vi "FTW-Connector-SendPoisonPill.vi"(0 "FTW Actor Connector":refnum<class "FTW-ActorConnector.lvclass">, 5 "Timeout":i32=100 format="%dmsec", 11 "error in":errorcluster) -> (4 "FTW Actor Connector out":refnum<class "FTW-ActorConnector.lvclass">, 6 "Response Header":string, 8 "Response Body":string, 10 "Timed out?":bool, 15 "error out":errorcluster)   [LabVIEW 2013, in "FTW-Actor.lvlib" / "FTW-ActorConnector.lvclass"]
uses:
  FTW-ActorConnector.lvclass
panel:
  # "Inputs"
  # "Outputs"
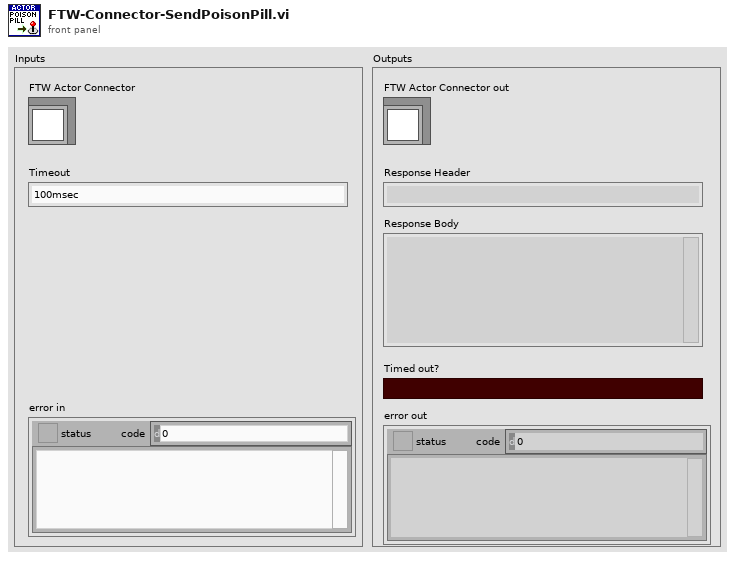
[diagram p1: front panel]
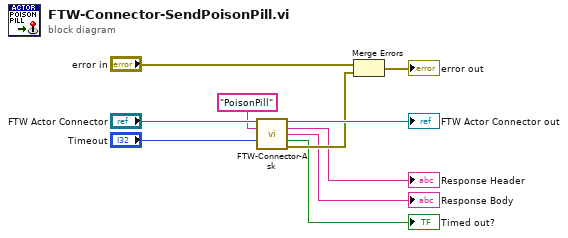
[diagram p0: block diagram]
diagram:
  n1 = call "FTW-Connector-Ask.vi"("FTW Actor Connector"="FTW Actor Connector", "Request Header"="PoisonPill" ("Message"), "Timeout"="Timeout") -> ("FTW Actor Connector out"=→"FTW Actor Connector out":refnum<class "FTW-ActorConnector.lvclass">, "Response Header"=→"Response Header":string, "Response Body"=→"Response Body":string, "Timed out?"=→"Timed out?":bool, "error out"=w5:errorcluster)  [unwired: 8 in]
  n2 = Merge Errors("error in", w5) -> (→"error out":errorcluster)
